vi "On Write Value.vi"(8 "error in (no error)":errorcluster, 11 "Proto Type Common in":refnum<class "Proto Type Common.lvclass">) -> (0 "error out":errorcluster, 3 "Proto Type Common out":refnum<class "Proto Type Common.lvclass">)   [LabVIEW 2020]
uses:
  Proto Type Common.lvclass
  Proto Type Common.lvclass/Proto Type Common.ctl
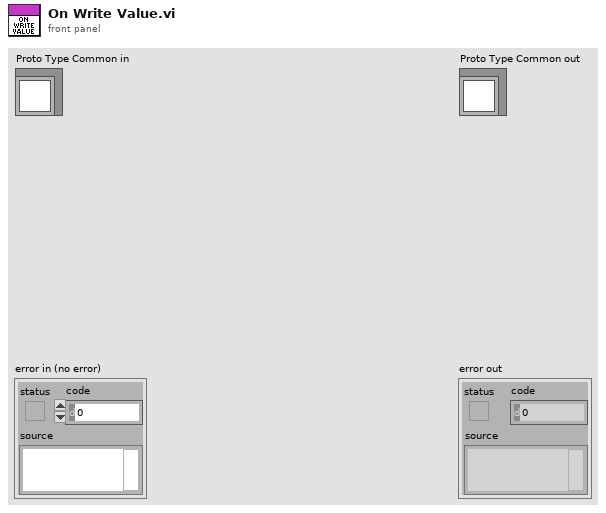
[diagram p1: front panel]
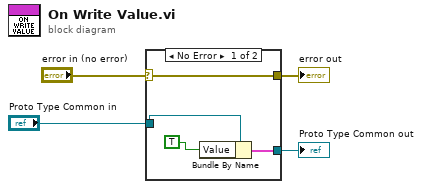
[diagram p0: block diagram]
diagram:
  n1 = case shown="No Error" "error in (no error)" {
    selector: "error in (no error)" -> [w7 w9]
    tunnel: "Proto Type Common in" -> [w8 w10]
    tunnel: [w6 w10] -> w3
    tunnel: [w7 w9] -> w1
    frame No Error {
      n2 = Bundle By Name(cluster=w8, "Value"=TRUE ("Value Set")) -> (w6:cluster{})
    }
    frame Error {
    }
  }
  "error out" <- w1
  "Proto Type Common out" <- w3
